vi "CarWash.vi"() -> ()   [LabVIEW 2018]
panel:
  in  "Vehicle Position":T1(radio)
  out "Car Wash Indicators":T2
  in  "stop":bool
  in  "Purchase Selection":cluster{"Deluxe Wash":bool, "Economy Wash":bool}
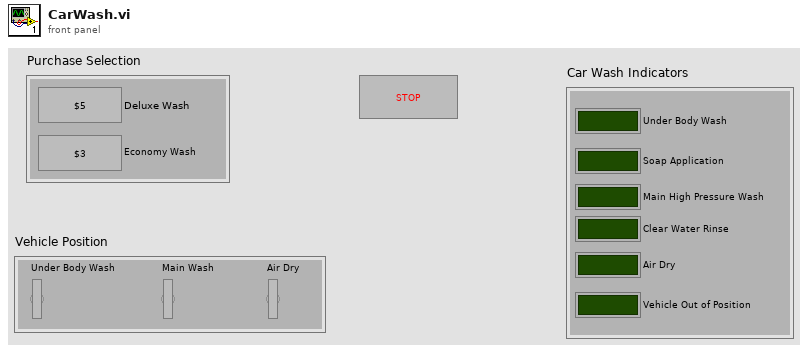
[diagram p1: front panel]
types:
  T1 = enum32{"Under Body Wash", "Main Wash", "Air Dry"}
  T2 = cluster{"Under Body Wash":bool, "Soap Application":bool, "Main High Pressure Wash":bool, "Clear Water Rinse":bool, "Air Dry":bool, "Vehicle Out of Position":bool}
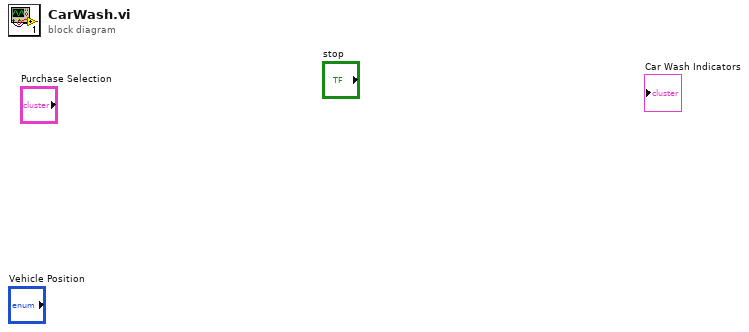
[diagram p0: block diagram]
diagram:
